vi "MRTCoilCurrentPWM.vi"(0 "DAQmx Task In":refnum<k21>="MRTCoilCurrentPWM", 4 "Current (% max)":dbl, 5 "Error In":errorcluster caption="error out") -> (14 "DAQmx Task Out":refnum<k21>="MRTCoilCurrentPWM", 15 "Period":dbl=0.022727272727272728, 16 "Pulse Width (s)":dbl=0.0012, 17 "Duty Cycle":dbl=0.05279999999999999, 19 "Error Out":errorcluster caption="error out")   [LabVIEW 2009]
uses:
  <vilib>/DAQmx/write.llb/DAQmx Write (Counter Frequency 1Chan 1Samp).vi
  Program Files (x86)/National Instruments/LabVIEW 2009/resource/objmgr/daqmx.rc
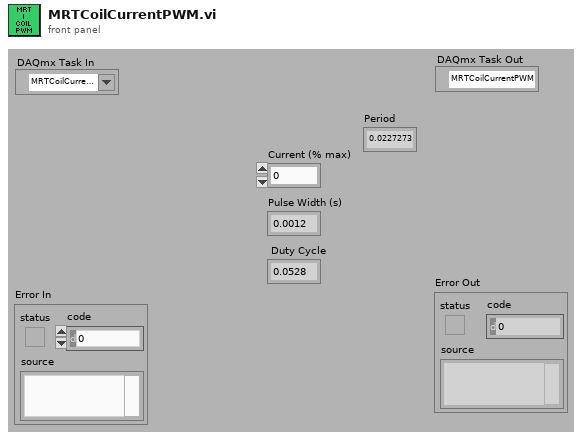
[diagram p1: front panel]
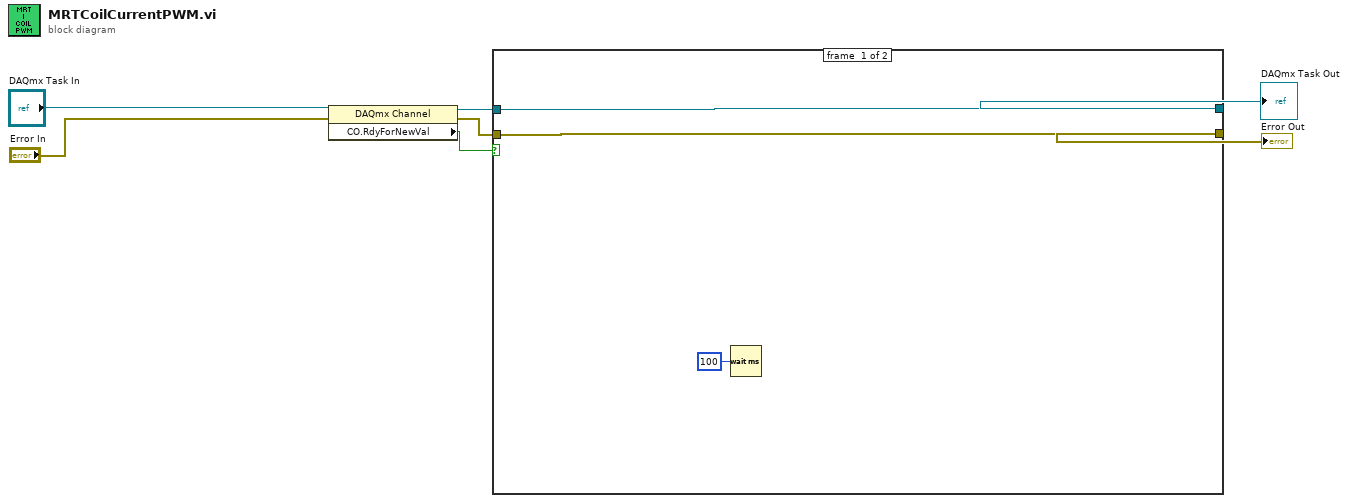
[diagram p0: block diagram]
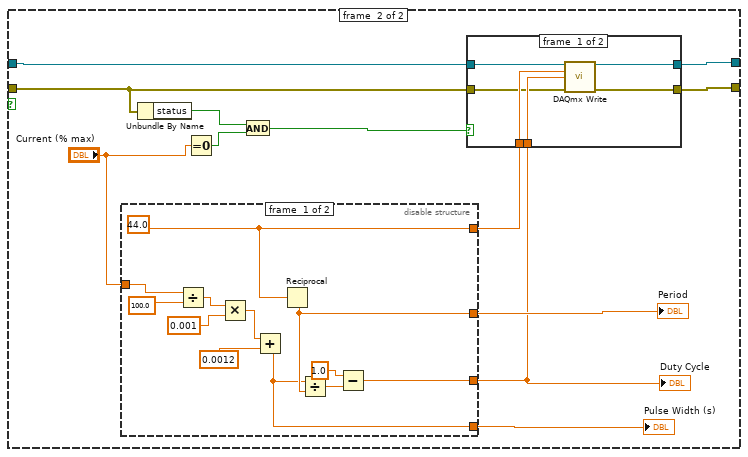
[diagram p2: hidden frame]
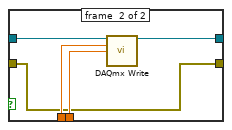
[diagram p3: hidden frame]
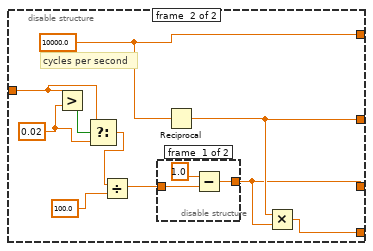
[diagram p4: hidden frame]
diagram:
  n1 = property class="DAQmx Channel"(reference="DAQmx Task In", error in="Error In") -> (reference out=w6:refnum<k21>, error out=w5:errorcluster, "CO.RdyForNewVal"=w7:bool)
  n2 = case shown="True" w7 {
    tunnel: w6 -> [w9 w22]
    tunnel: w5 -> [w8 w15]
    tunnel: [w9 w21] -> w4
    tunnel: [w8 w20] -> w1
    frame #0 {
      n3 = Wait (ms)(milliseconds to wait=u32 100) -> ()  [unwired: 1 out]
    }
    frame #1 {
      n4 = disable-structure shown="Enabled" {
        disable-tunnel: [w42 w55] -> w19
        disable-tunnel: [w41 w52] -> w18
        disable-tunnel: [w40 w50] -> w17
        disable-tunnel: "Current (% max)" -> [w38 w48]
        disable-tunnel: [w34 w51] -> w16
        frame #0 {
          w42 = 44.0 ("Frequency (Hz)")
          n5 = Divide(x=w38, y=100.0 ("Current (% max) 2")) -> (x/y=w39:dbl)
          n6 = Multiply(x=w39, y=0.001 ("100% Width")) -> (x*y=w44:dbl)
          n7 = Add(x=w44, y=0.0012 ("PWM Center Width")) -> (x+y=w40:dbl)
          n8 = Reciprocal(x=w42) -> (1/x=w41:dbl)
          n9 = Divide(x=w40, y=w41) -> (x/y=w35:dbl)
          n10 = Subtract(x=1.0, y=w35) -> (x-y=w34:dbl)
        }
        frame #1 {
          w47 = 0.02
          w55 = 10000.0
          # "cycles per second"
          n11 = Greater?(x=w48, y=w47) -> (0:w49:bool)
          n12 = Select(t=w48, s=w49, f=w47) -> (s? t:f=w46:dbl)
          n13 = Divide(x=w46, y=100.0) -> (x/y=w53:dbl)
          n14 = disable-structure shown="Enabled" {
            disable-tunnel: w53 -> [w58 w59]
            disable-tunnel: [w56 w59] -> w51
            frame #0 {
              n15 = Subtract(x=1.0, y=w58) -> (x-y=w56:dbl)
            }
            frame #1 {
            }
          }
          n16 = Reciprocal(x=w55) -> (1/x=w52:dbl)
          n17 = Multiply(x=w52, y=w51) -> (x*y=w50:dbl)
        }
      }
      "Duty Cycle" <- w16
      "Pulse Width (s)" <- w17
      "Period" <- w18
      n18 = Unbundle By Name(w15) -> ("status"=w14:bool)
      n19 = Equal To 0?(x="Current (% max)") -> (x = 0?=w12:bool)
      n20 = And(x=w14, y=w12) -> (x .and. y?=w11:bool)
      n21 = case shown="False" w11 {
        tunnel: w22 -> [w28 w33]
        tunnel: w15 -> [w23 w29]
        tunnel: [w27 w32] -> w21
        tunnel: [w24 w29] -> w20
        tunnel: w19 -> [w26 w31]
        tunnel: w16 -> [w25 w30]
        frame #0 {
          n22 = call-poly <vilib>:"DAQmx Write.vi"("task/channels in"=w28, "frequency"=w26, "duty cycle"=w25, "error in"=w23) -> ("task out"=w27:refnum<k21>, "error out"=w24:errorcluster)  [unwired: 9 in, 1 out]
        }
        frame #1 {
          n23 = call-poly <vilib>:"DAQmx Write.vi"("task/channels in"=w33, "frequency"=w31, "duty cycle"=w30) -> ("task out"=w32:refnum<k21>)  [unwired: 10 in, 2 out]
        }
      }
    }
  }
  "DAQmx Task Out" <- w4
  "Error Out" <- w1
